vi "Make single scan multivariable file.vi"() -> ()   [LabVIEW 2013]
uses:
  scan parameters.ctl
  <vilib>/Analysis/1siggen.llb/Ramp Pattern by Delta.vi
  <vilib>/Analysis/polynomials.llb/1D Polynomial Evaluation (DBL).vi
  <vilib>/Analysis/NI_AALBase.lvlib
  <vilib>/Analysis/NI_AALPro.lvlib
panel:
  in  "P(x) 3":dbl[](array[numeric])=[11.3933866, 0.0219842824, -0.00436825015] caption="P(x) ascending order of power." min=0.0 max=127.0 format="%#.6f"
  in  "P(x) 2":dbl[](array[numeric])=[9.48225287, 0.261028858, -0.0092426937] caption="42 torr he\\n2" min=0.0 max=127.0 format="%#.6f"
  in  "P(x)":dbl[](array[numeric])=[11.8886568, -0.11977964, -0.00212912113] caption="P(x) ascending order of power." min=0.0 max=127.0 format="%#.6f"
  in  "equation for vals 2":bool=TRUE
  in  "precision (12) 2":i16=12
  in  "precision (12)":i16=12
  in  "2D scan details":T2(array[cluster])=[{"Scan parameters"={"Scan Start"=25.2, "Scan End"=15.8, "Scan Step Size"=-1.0, "# Shots Each Step"=20, "single direction?"=TRUE}, "device and variable preamble"="Device = \"PL1-PresCtrl-Low1,PlasmaLensLowPressureControl\"\nVariable = \"P. Control Up (Torr),pressure\""}, {"Scan parameters"={"Scan Start"=32.0, "Scan End"=17.0, "Scan Step Size"=-0.25, "# Shots Each Step"=5, "single direction?"=TRUE}, "device and variable preamble"="Device = \"PL1-PresCtrl-Low1\"\nVariable = \"P. Control Up (Torr)\""}] {"Scan parameters"."Scan Start" format="%#.9p"; "Scan parameters"."Scan End" format="%#.9p"; "Scan parameters"."Scan Step Size" format="%#.9p"}
  out "spreadsheet string":string="[Scan1]\r\nDevice = \"PL1-PresCtrl-Low1,PlasmaLensLowPressureControl\"\nVariable = \"P. Control Up (Torr),pressure\"\r\nValues:#shots = \"(25.200000000000,7.518133):20|(24.200000000000,7.743091):20|(23.200000000000,7.963791):20|(22.200000000000,8.180233):20|(21.200000000000,8.392416):20|(20.200000000000,8.600341):20|(19.200000000000,8.804008):20|(18.200000000000,9.003417):20|(17.200000000000,9.198568):20|(16.200000000000,9.389460):20\""
  # "Instructions:\nOption 1: Use only the first scan parameters and set equation for vals to true. Then enter the polynomials.\nIn this case, eg set device and variable preamble are... Device = \"PL1-PresCtrl-Low1,PlasmaLensLowPressureControl\"\nVariable = \"P. Control Up (Torr),pressure\"\nOption 2: Use both scan parameter clusters"
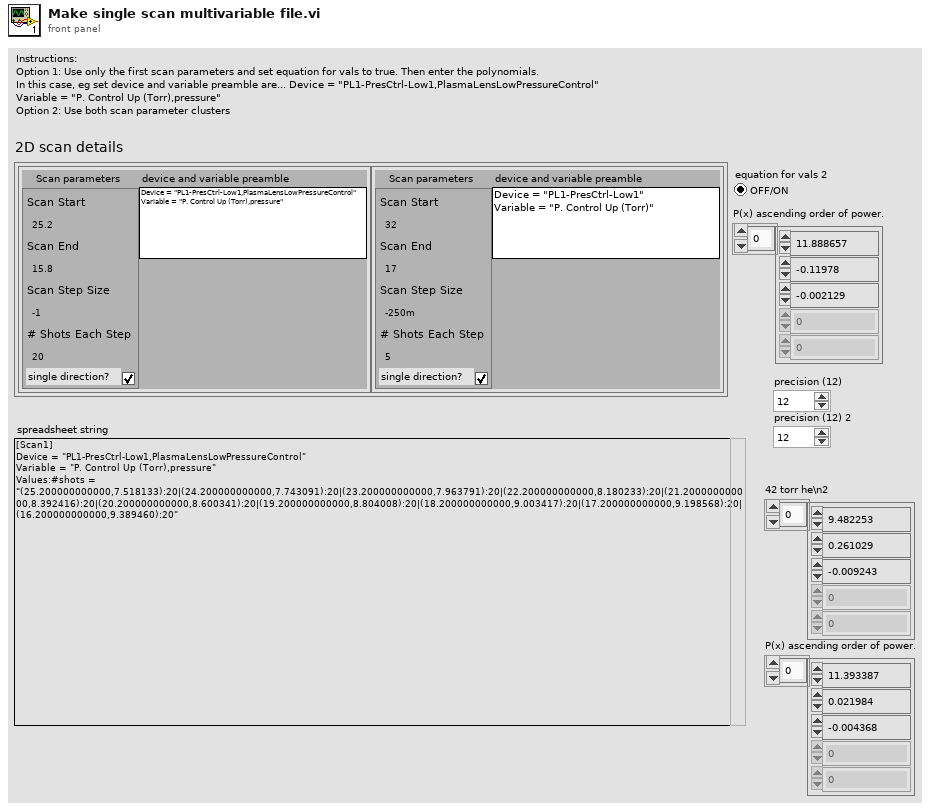
[diagram p1: front panel]
types:
  T1 = typedef "scan parameters.ctl" = cluster{"Scan Start":dbl, "Scan End":dbl, "Scan Step Size":dbl, "# Shots Each Step":u32, "single direction?":bool}
  T2 = cluster{"Scan parameters":T1, "device and variable preamble":string}[]
  T3 = cluster{"Scan parameters":T1, "device and variable preamble":string}
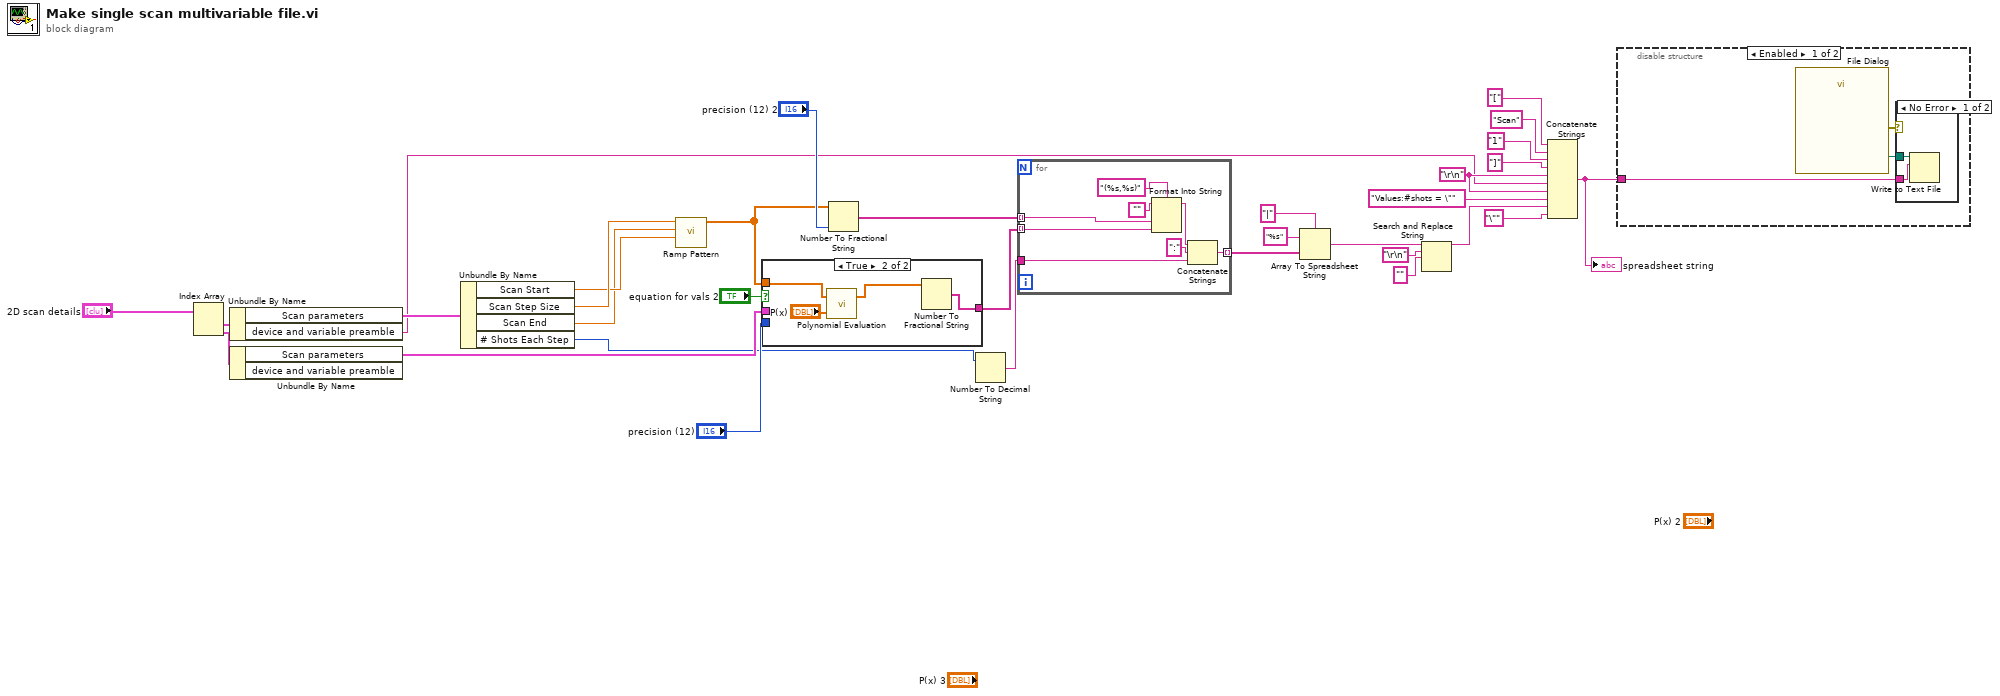
[diagram p0: block diagram]
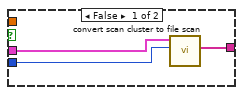
[diagram p2: hidden frame]
diagram:
  w27 = "\r\n"
  n1 = Index Array(array="2D scan details") -> (element #1=w31:T3, element #2=w30:T3)  [unwired: 2 in]
  n2 = Unbundle By Name(w31) -> ("Scan parameters"=w7:T1, "device and variable preamble"=w4:string)
  n3 = Unbundle By Name(w30) -> ("Scan parameters"=w29:T1)  [unwired: 1 out]
  n4 = Unbundle By Name(w7) -> ("Scan Start"=w19:dbl, "Scan Step Size"=w20:dbl, "Scan End"=w18:dbl, "# Shots Each Step"=w16:u32)
  n5 = call-poly <vilib>:"Ramp Pattern.vi"("start"=w19, "end"=w18, "delta"=w20) -> ("Ramp Pattern"=w2:dbl[])  [unwired: 6 in, 2 out]
  n6 = case shown="True" "equation for vals 2" {
    tunnel: w29 -> [w35 _]
    tunnel: "precision (12)" -> [w34 _]
    tunnel: [w33 w36] -> w6
    tunnel: w2 -> [_ w39]
    frame False {
      n7 = call "convert scan cluster to file scan.vi"("precision (12)"=w34, "Scan parameters"=w35) -> ("values"=w33:string[])  [unwired: 7 in, 2 out]
    }
    frame True {
      n8 = call-poly <vilib>:"Polynomial Evaluation.vi"("P(x)"="P(x)", "A"=w39) -> ("P(A)"=w37:dbl[])  [unwired: 1 out]
      n9 = Number To Fractional String(number=w37) -> (F-format string=w36:string[])  [unwired: 3 in]
    }
  }
  n10 = Number To Fractional String(number=w2, precision (6)="precision (12) 2") -> (F-format string=w11:string[])  [unwired: 2 in]
  n11 = Number To Decimal String(number=w16) -> (decimal integer string=w15:string)  [unwired: 1 in]
  n12 = for {
    tunnel: w11 -> [w42] mode=indexing
    tunnel: w15 -> [w46]
    tunnel: [w45] -> w14 mode=indexing
    tunnel: w6 -> [w41] mode=indexing
    n13 = Format Into String(format string="(%s,%s)", initial string="", w42, w41) -> (resulting string=w40:string)  [unwired: 1 in, 1 out]
    n14 = Concatenate Strings(w40, ":" ("string"), w46) -> (w45:string)
  }
  n15 = Array To Spreadsheet String(delimiter (Tab)="|", array=w14, 3:"%s" ("format string")) -> (spreadsheet string=w10:string)
  n16 = Search and Replace String(input string=w10, search string="\r\n", replace string="" ("replace string (\"\")")) -> (result string=w5:string)  [unwired: 5 in, 3 out]
  n17 = Concatenate Strings("[" ("string"), "Scan", "1" ("scan #"), "]" ("string"), w27, w4, w27, "Values:#shots = \"" ("string"), w5, "\"" ("string")) -> (w1:string)
  "spreadsheet string" <- w1
  n18 = disable-structure shown="Enabled" {
    disable-tunnel: w1 -> [w48 _]
    frame Enabled {
      n19 = call "File Dialog"() -> ("selected path"=w49:path, "error out"=w50:errorcluster)  [unwired: 12 in, 2 out]
      n20 = case shown="No Error" w50 {
        tunnel: w48 -> [w52 _]
        tunnel: w49 -> [w51 _]
        frame No Error {
          n21 = Write to Text File(file (use dialog)=w51, text=w52) -> ()  [unwired: 2 in, 3 out]
        }
        frame Error {
        }
      }
    }
    frame Disabled {
    }
  }
